vi "Configure SmtpEmail.vi"(5 "Port":i32=25, 6 "Enable SSL":bool=TRUE, 7 "SMTP Outgoing Mail Server":string="smtp.gmail.com", 8 "error in (no error)":errorcluster, 9 "Email Account Password":string="1110810220", 10 "Email Account ID":string="qianlingf@gmail.com", 11 "StmpEmail in":refnum<class "StmpEmail.lvclass">) -> (0 "error out":errorcluster, 3 "StmpEmail out":refnum<class "StmpEmail.lvclass">)   [LabVIEW 2015, in "StmpEmail.lvclass"]
uses:
  StmpEmail.lvclass
  StmpEmail.lvclass/StmpEmail.ctl
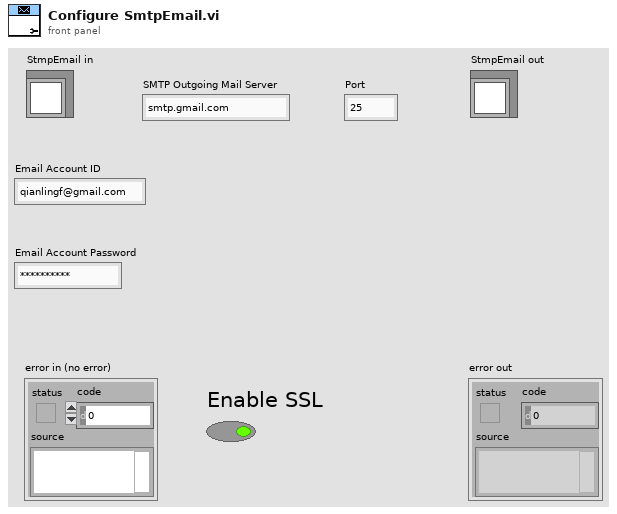
[diagram p1: front panel]
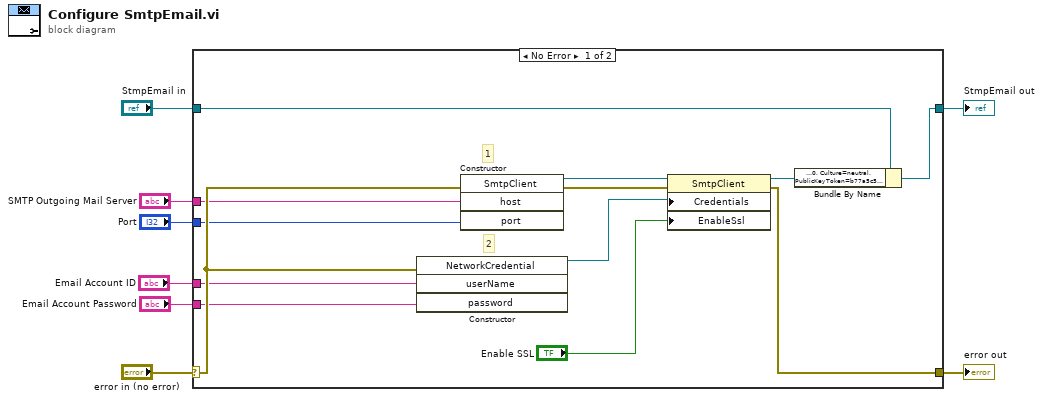
[diagram p0: block diagram]
diagram:
  n1 = case shown="No Error" "error in (no error)" {
    selector: "error in (no error)" -> [w17 w23]
    tunnel: [w12 w23] -> w7
    tunnel: [w9 w22] -> w5
    tunnel: "StmpEmail in" -> [w11 w22]
    tunnel: "SMTP Outgoing Mail Server" -> [w16 _]
    tunnel: "Port" -> [w15 _]
    tunnel: "Email Account ID" -> [w14 _]
    tunnel: "Email Account Password" -> [w13 _]
    frame No Error {
      # "2"
      # "1"
      n2 = constructor class="NetworkCredential"(error in=w17, "userName"=w14, "password"=w13) -> (reference out=w18:refnum<k24>)  [unwired: 2 in, 4 out]
      n3 = constructor class="SmtpClient"(error in=w17, "host"=w16, "port"=w15) -> (reference out=w21:refnum<k24>, error out=w19:errorcluster)  [unwired: 2 in, 3 out]
      n4 = property class="SmtpClient"(reference=w21, error in=w19, "Credentials"=w18, "EnableSsl"="Enable SSL") -> (reference out=w10:refnum<k24>, error out=w12:errorcluster)
      n5 = Bundle By Name(cluster=w11, "SmtpEamil Ref"=w10) -> (w9:refnum<class "StmpEmail.lvclass">)
    }
    frame Error {
    }
  }
  "error out" <- w7
  "StmpEmail out" <- w5
